vi "writeToXML.vi"(8 "error in (no error)":errorcluster, 10 "ClassLabel":string, 11 "TCSAtmosphericDispersionCommand in":refnum<class "TCSAtmosphericDispersionCommand.lvclass">) -> (0 "error out":errorcluster, 2 "XML out":string, 3 "TCSAtmosphericDispersionCommand out":refnum<class "TCSAtmosphericDispersionCommand.lvclass">)   [LabVIEW 2022 SP3, in "TCSDataDefinitions.lvlib" / "TCSAtmosphericDispersionCommand.lvlib" / "TCSAtmosphericDispersionCommand.lvclass"]
uses:
  TCSAtmosphericDispersionCommand.lvclass
  TCSCommand/TCSCommand/TCSCommand.lvclass
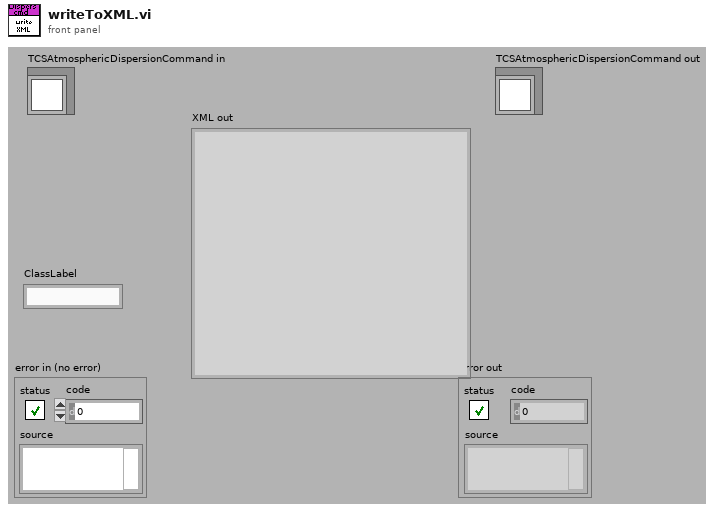
[diagram p1: front panel]
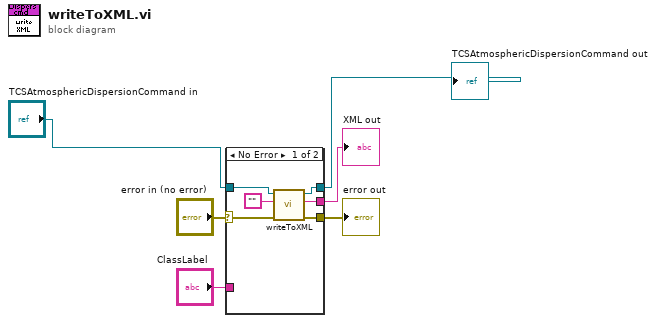
[diagram p0: block diagram]
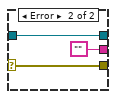
[diagram p2: hidden frame]
diagram:
  n1 = case shown="No Error" "error in (no error)" {
    selector: "error in (no error)" -> [w11 w15]
    tunnel: [w10 w15] -> w5
    tunnel: [w8 w14] -> w1
    tunnel: "TCSAtmosphericDispersionCommand in" -> [w9 w14]
    tunnel: [w7 ""] -> w4
    tunnel: "ClassLabel" -> [_ _]
    frame No Error {
      n2 = call-parent "writeToXML.vi"("error in (no error)"=w11, "Class Label"="", "TCSCommand in"=w9) -> ("error out"=w10:errorcluster, "XML out"=w7:string, "TCSCommand out"=w8:refnum<class "TCSAtmosphericDispersionCommand.lvclass">)  [unwired: 6 in]
    }
    frame Error {
    }
  }
  "error out" <- w5
  "XML out" <- w4
  "TCSAtmosphericDispersionCommand out" <- w1
